vi "Module Type.vi"(11 "GenericGuiDI in":refnum<class "GenericGuiDI.lvclass">) -> (2 "Module Type":string)   [LabVIEW 2020, in "VolatusDAQGenericGUI.lvlib" / "GenericGuiDI.lvclass"]
uses:
  GenericGuiDI.lvclass
  GenericGuiDI.lvclass/GenericGuiDI.ctl
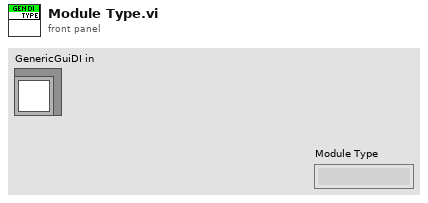
[diagram p1: front panel]
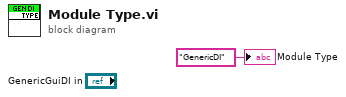
[diagram p0: block diagram]
diagram:
  "Module Type" <- "GenericDI" ("Module Type")
